vi "ReadProjectData.vi"(8 "error in (no error)":errorcluster, 11 "Project.lvclass In":refnum<class "Project.lvclass">) -> (0 "error out":errorcluster, 2 "ProjectDataTable":T1, 3 "Project.lvclass Out":refnum<class "Project.lvclass">)   [LabVIEW 2014, in "Project.lvclass"]
uses:
  Project.lvclass
  ProjectDataTableTypeDefine.ctl
  Project.lvclass/Project.ctl
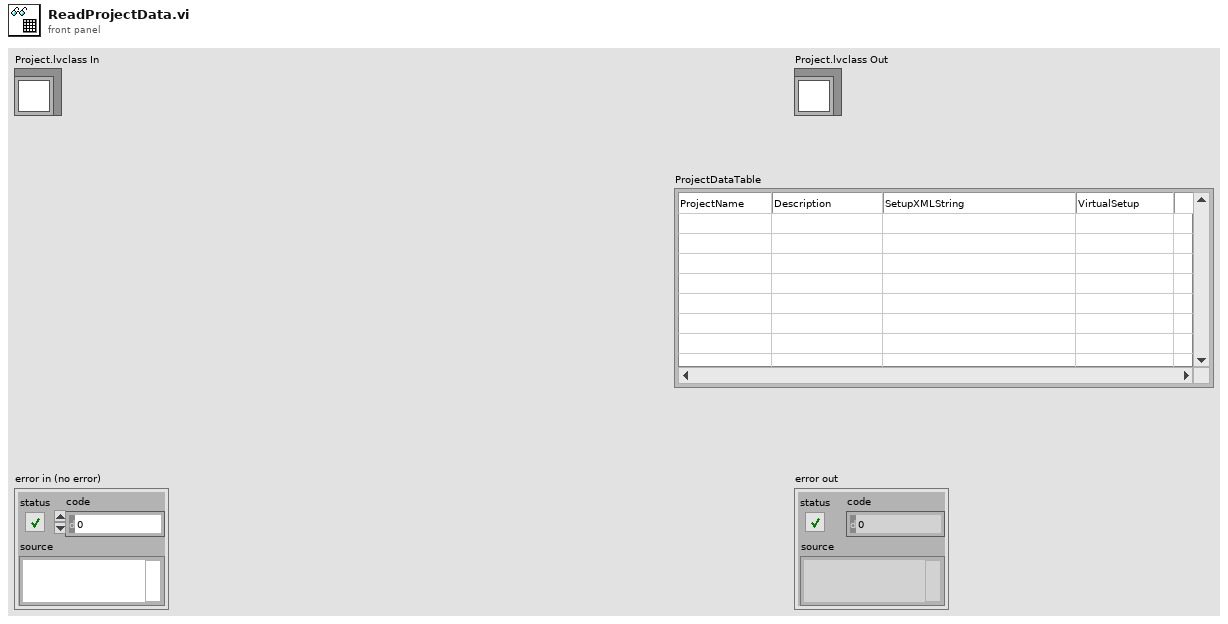
[diagram p1: front panel]
types:
  T1 = typedef "Project.lvclass/ProjectDataTableTypeDefine.ctl" = string[][]
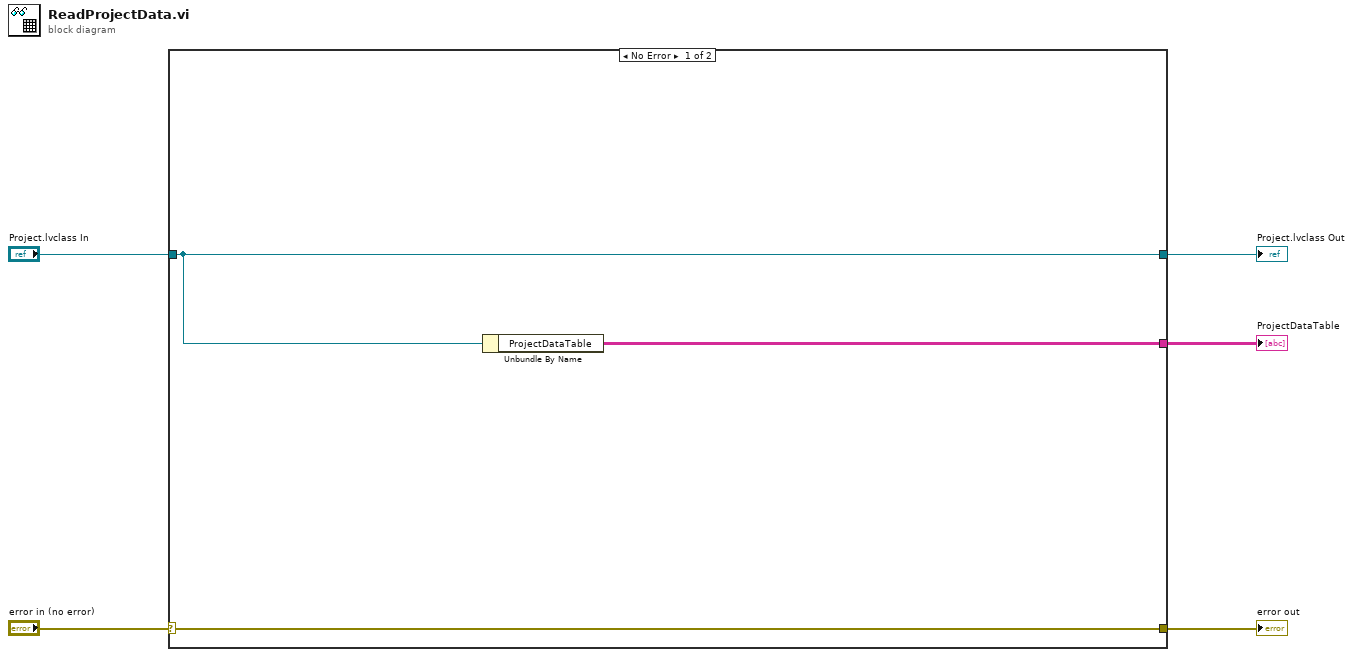
[diagram p0: block diagram]
diagram:
  n1 = case shown="No Error" "error in (no error)" {
    selector: "error in (no error)" -> [w8 w10]
    tunnel: [w8 w10] -> w4
    tunnel: "Project.lvclass In" -> [w7 w9]
    tunnel: [w7 w9] -> w2
    tunnel: [w6 _] -> w1
    frame No Error {
      n2 = Unbundle By Name(w7) -> ("ProjectDataTable"=w6:T1)
    }
    frame Error {
    }
  }
  "error out" <- w4
  "Project.lvclass Out" <- w2
  "ProjectDataTable" <- w1
